vi "Check if controls or constants.vi"() -> (3 "Controls or Constants":T1)   [LabVIEW 2016, in "PantherLAB_Scripting.lvlib"]
uses:
  PantherLAB_Scripting.lvlib
  Controls or Constants--enum.ctl
  <resource>/dialog/lvconfig.llb/LV Config Read Numeric (I32).vi
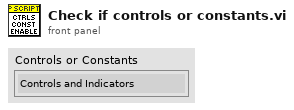
[diagram p1: front panel]
types:
  T1 = typedef "PantherLAB_Scripting.lvlib/Controls or Constants--enum.ctl" = enum16{"Controls and Indicators", "Constants and Indicators"}
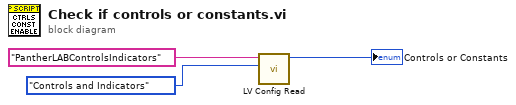
[diagram p0: block diagram]
diagram:
  n1 = call-poly <resource>:"LV Config Read.vi"("default value"=Controls_or_Constants--enum."Controls and Indicators" ("Create"), "key"="PantherLABControlsIndicators") -> ("value"=→"Controls or Constants":i32)  [unwired: 3 in, 2 out]
